vi "DAC_wait_end-of-move.vi"(11 "FPGA VI Reference In":T1) -> (3 "FPGA VI Reference Out":T1)   [LabVIEW 2013]
uses:
  fpga-bitfile-ref.ctl
  <vilib>/Utility/error.llb/Error Cluster From Error Code.vi
  <vilib>/rvi/errors/niLvFpgaAdjustHostInterfaceError.vi
  <vilib>/rvi/interface/nirviReadWriteControl/nirviReadWriteControl.xnode
  FPGA Bitfiles/fpgabatch18_sbRIO9612RIO0_FPGAMAINlock-in_BbNldMosBaM.lvbitx
  NiFpgaLv.dll
panel:
  out "error out":errorcluster
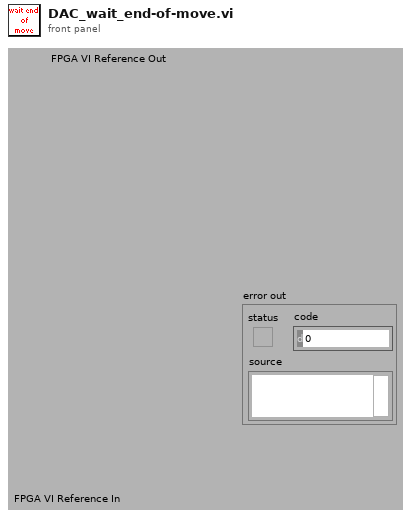
[diagram p1: front panel]
types:
  T1 = typedef "fpga-bitfile-ref.ctl" = refnum<k20>
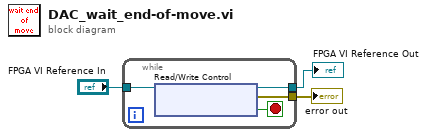
[diagram p0: block diagram]
diagram:
  n1 = while {
    tunnel: [w7] -> w2
    tunnel: [w6] -> w1
    tunnel: "FPGA VI Reference In" -> [w5]
    stop <- w4 stop-if-true
    n2 = xnode "Read/Write Control"("FPGA VI Reference In"=w5) -> ("FPGA VI Reference Out"=w7:T1, "error out"=w6:errorcluster, "move bus ready"=w4:bool)  [unwired: 1 in]
  }
  "error out" <- w1
  "FPGA VI Reference Out" <- w2
